vi "Control de Temperatura.vi"() -> ()   [LabVIEW 2019]
panel:
  in  "RATA DE T° (5°C/Seg)":dbl(knob) scale=0.0..10.0
  in  "Selector":bool
  out "Sensor de Temperatura":i32(slide) scale=0.1..100.0
  # "Incrementar"
  # "Decrementar"
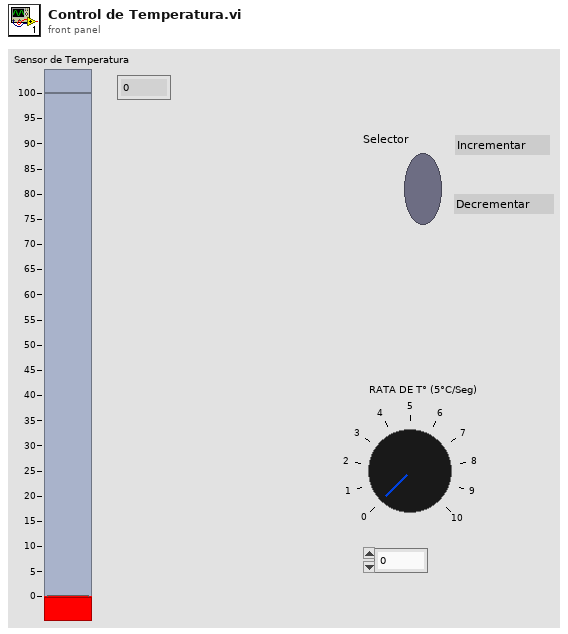
[diagram p1: front panel]
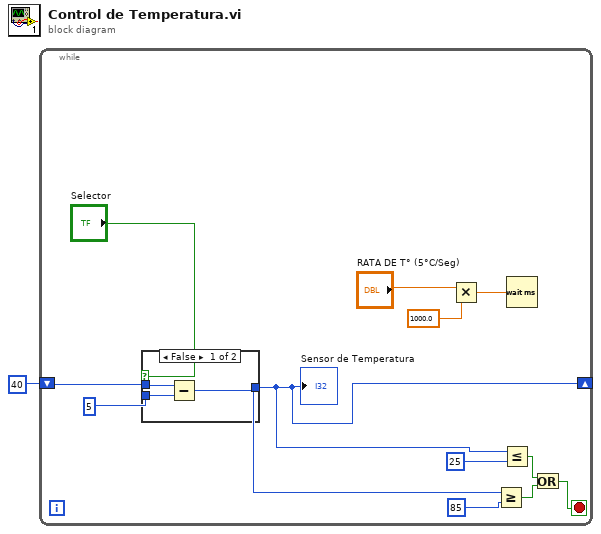
[diagram p0: block diagram]
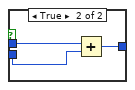
[diagram p2: hidden frame]
diagram:
  n1 = while {
    shift-right: [w3] -> _
    shift-left: 40 -> [w5]
    stop <- w13 stop-if-true
    n2 = case shown="False" "Selector" {
      tunnel: w5 -> [w15 w19]
      tunnel: 5 ("y") -> [w14 w18]
      tunnel: [w16 w17] -> w3
      frame False {
        n3 = Subtract(x=w15, y=w14) -> (x-y=w16:i32)
      }
      frame True {
        n4 = Add(x=w19, y=w18) -> (x+y=w17:i32)
      }
    }
    "Sensor de Temperatura" <- w3
    n5 = Multiply(x="RATA DE T° (5°C/Seg)", y=1000.0) -> (x*y=w6:dbl)
    n6 = Greater Or Equal?(x=w3, y=85) -> (x >= y?=w11:bool)
    n7 = Less Or Equal?(x=w3, y=25) -> (x <= y?=w12:bool)
    n8 = Wait (ms)(milliseconds to wait=w6) -> ()  [unwired: 1 out]
    n9 = Or(x=w12, y=w11) -> (x .or. y?=w13:bool)
  }
